vi "Spectrometer - Test activeX.vi"() -> ()   [LabVIEW 2014]
uses:
  NGSLabspec/NGSLabSpec.llb/MoveMotor Mode.ctl
  NGSLabspec/NGSLabSpec.llb/MoveMotor Motor Name.ctl
  NGSLabspec/NGSLabSpec.llb/GetMotorPosition Mode.ctl
  NGSLabspec/NGSLabSpec.llb/Acquire Mode.ctl
  NGSLabspec/NGSLabSpec.llb/GetValue Mode.ctl
  NGSLabspec/NGSLabSpec.llb/PutValue Name.ctl
  NGSLabspec/NGSLabSpec.llb/Template Mode.ctl
  NGSLabspec/NGSLabSpec.llb/Template Parameter.ctl
  NGSLabspec/NGSLabSpec.llb/GetMotorPosition Label Option.ctl
  NGSLabspec/NGSLabSpec.llb/Exec Command.ctl
panel:
  in  "stop":bool
  in  "OK Button":bool
  out "DataID":i32
  in  "Function":T1(tab)
  out "Array":i32[](array[numeric])
  in  "GetValue Mode":T2
  out "Value":variant
  in  "pValue":variant
  in  "Name":T3
  in  "Acquisition Mode":T4 items=["Spectrum", "Image", "Spectrum (Labspec Parameters)", "Spectral Image", "Get Detector Temperature", "Real Time Acquisition", "Set Photomultiplier Parameter", "Macro Spot", "Cancel Acquisition", "Set Detector"]
  in  "From (nm)":dbl=1.0
  in  "To (nm)":dbl=1.0
  in  "Integration Time (s)":dbl=1.0
  in  "Number of Accumulations":i32
  out "Acq":i32
  in  "Mode":T5 items=["Value"=0, "Step"=1, "Index"=2, "String"=3, "Calibrate"=4, "Origin"=5, "Stop"=6, "Value to Step"=7, "No Wait"=10, "No Message"=100]
  in  "Motor Name":T6=enum."Hole"
  in  "Position Value":dbl=1.0
  in  "Position Name":string
  out "MoveID":i32
  in  "Mode":T7 items=["Value", "Step", "Index", "Size", "Full Size"]
  in  "Motor Name":T6
  out "Position":string
  in  "Label Option":T8 items=[""=0, "Index to Value"=10, "Index to String"=20, "Full Index to Value"=30, "Full Index to String"=40]
  out "pValue Out":variant
  in  "Template Mode":T9
  in  "Template Parameter":T10
  in  "Template Name":string
  in  "Template Value":variant
  out "error out":errorcluster
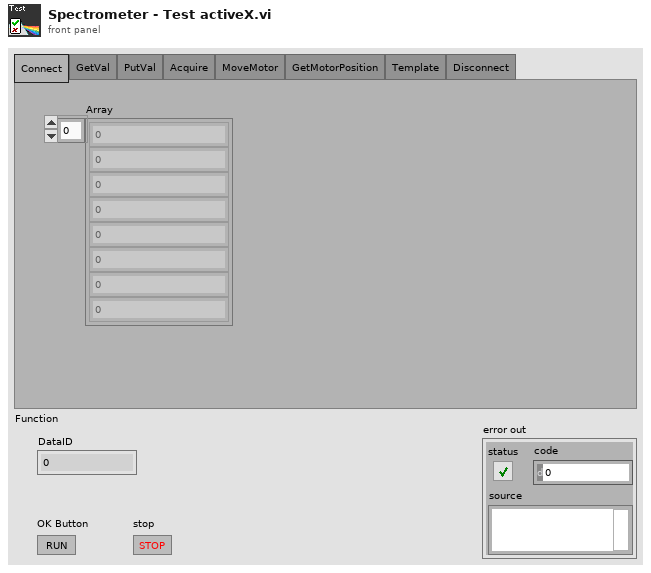
[diagram p1: front panel]
types:
  T1 = enum32{"Connect", "GetVal", "PutVal", "Acquire", "MoveMotor", "GetMotorPosition", "Template", "Disconnect"}
  T2 = typedef "GetValue Mode.ctl" = enum16{"XY Data", "Data", "MapPoint: Spectrum Index", "Axis Labels", "Axis Units", "Axis", "Axis Index", "Axis Size", "Axis Type", "Intensity", "Frequency", "X", "Y", "Z", "Time", "Double Cursor", "Pointer Limits", "Active Cursors", "Nearest Axis Index", "Acquisition Information", "Custom Information", "History Information", "Data Name", "Dispersion", "Dispersion Parameters", "Labspec Path", "User Level", "System Name", "Autofocus Diode", "Exposure Time", "Live Time", "Labspec Accumulation", "Alignment Diode"}
  T3 = typedef "PutValue Name.ctl" = enum16{"XY Data", "Data", "MapPoint:SpectrumIndex", "Axis Labels", "Axis Units", "Axis", "Axis Limits", "Frequency Unit", "Intensity Unit", "Cursor Type", "Pointer Limits", "Active Cursors", "Special Script Type", "CCD Shutter", "Laser", "SWIFT", "Labspec Exposure Time", "Labspec Accumulation", "Active Frame"}
  T4 = typedef "Acquire Mode.ctl" = u16
  T5 = typedef "MoveMotor Mode.ctl" = u16
  T6 = typedef "MoveMotor Motor Name.ctl" = enum16{"Spectro", "Premono", "Grating", "Slit", "Hole", "X", "Y", "XT", "YT", "XL", "YL", "Z", "Laser", "Filter", "Objective", "Detector", "Detector Temperature"}
  T7 = typedef "GetMotorPosition Mode.ctl" = u16
  T8 = typedef "GetMotorPosition Label Option.ctl" = u16
  T9 = typedef "Template Mode.ctl" = enum16{"Load", "Save", "Add To List", "Set Value", "Get Value", "Apply ", "Get Status", "Save Current Config", "Test", "Apply No Spectro"}
  T10 = typedef "Template Parameter.ctl" = enum16{"Laser", "Filter", "Accumulation", "Spike", "Auto Exposure", "Auto Focus", "Grating", "Raman Polarizer", "Laser Polarizer", "Central Position", "Position From", "Position To", "Exposition", "Hole", "Slit", "AutoExposure Min", "AutoExposure Max", "Extended Range", "Objective"}
  T11 = enum16{"Generic Data", "Spectrum", "Spectral Profile Image", "Map", "Video", "First Data", "Next Data"}
  T12 = typedef "Exec Command.ctl" = u16
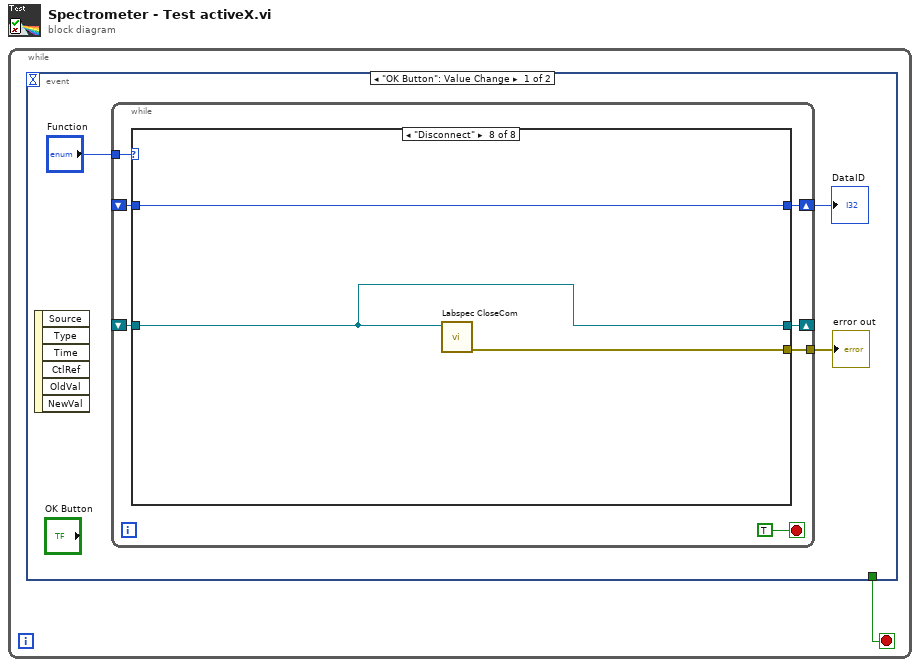
[diagram p0: block diagram]
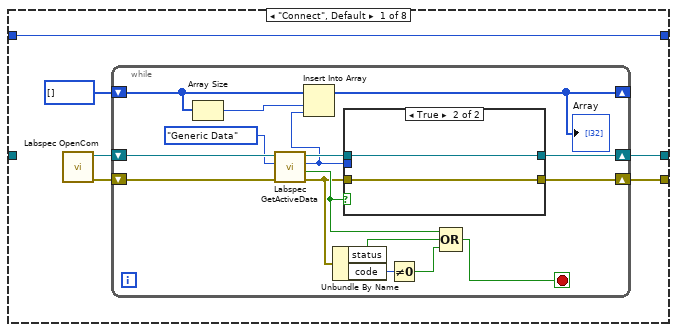
[diagram p2: hidden frame]
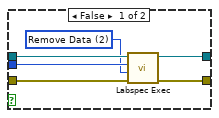
[diagram p3: hidden frame]
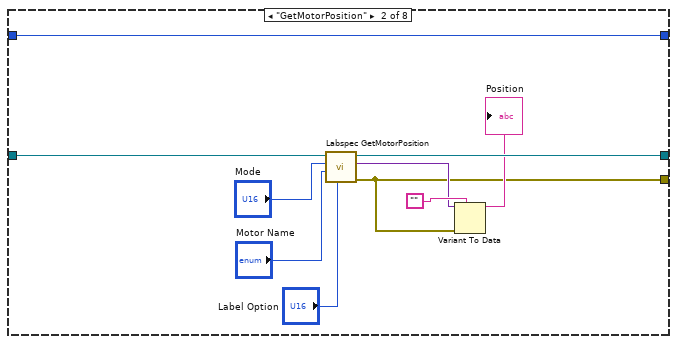
[diagram p4: hidden frame]
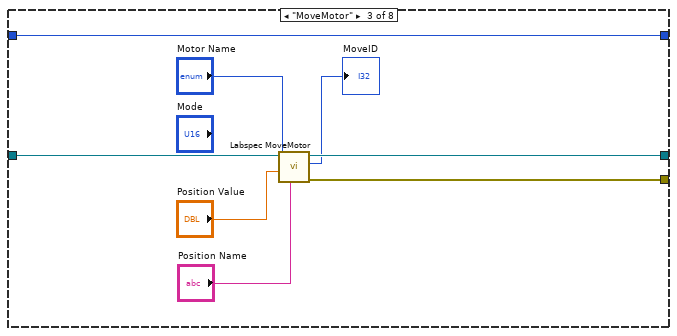
[diagram p5: hidden frame]
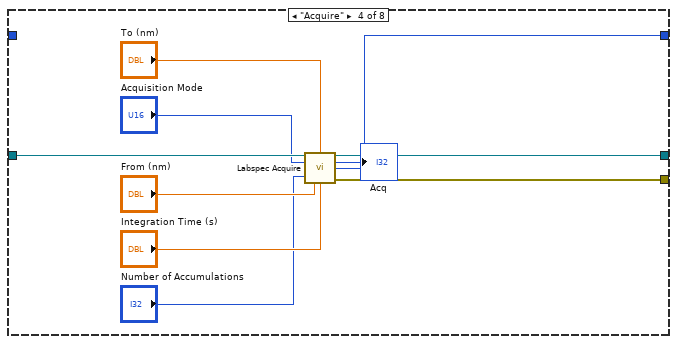
[diagram p6: hidden frame]
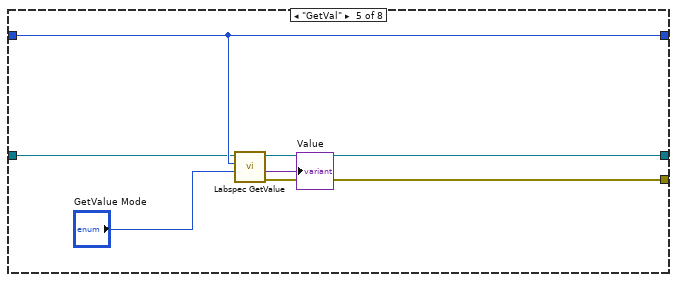
[diagram p7: hidden frame]
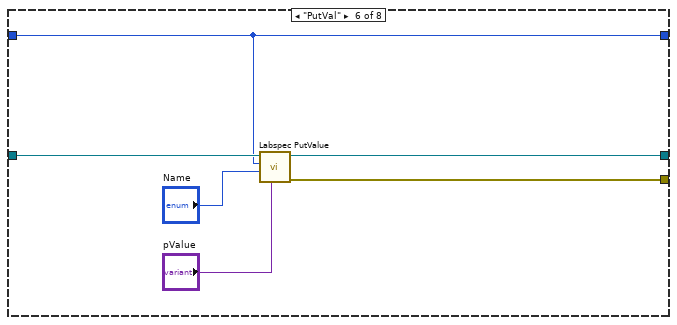
[diagram p8: hidden frame]
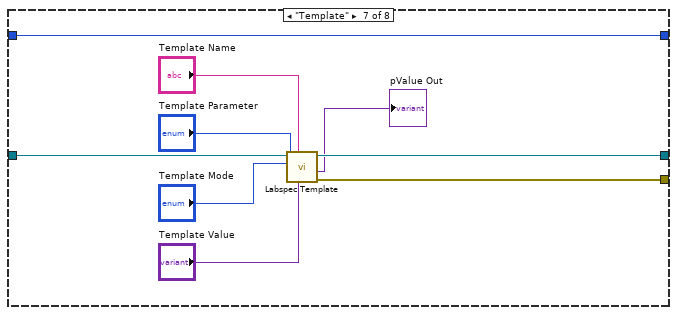
[diagram p9: hidden frame]
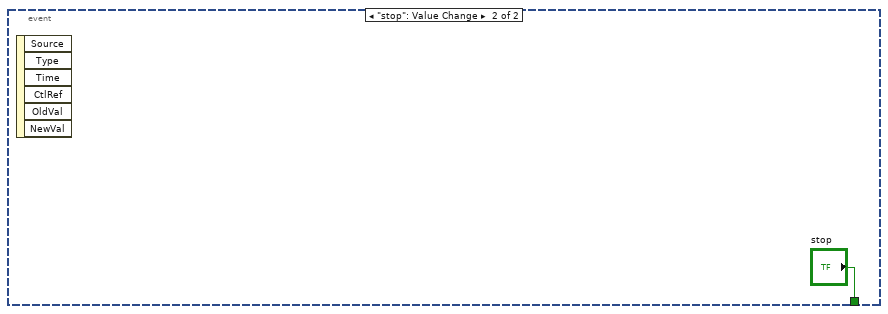
[diagram p10: hidden frame]
diagram:
  n1 = while {
    stop <- w1 stop-if-true
    n2 = event shown="[0] \"OK Button\": Value Change" {
      selector: _ -> [_ _]
      dyn-events: _ -> [_ _]
      timeout: _ -> [_ _]
      tunnel: [_ "stop"] -> w1
      event "OK Button": Value Change {
        n3 = event-data() -> ()  [unwired: 1 in, 6 out]
        n4 = while {
          shift-right: [w11] -> _
          shift-left: _ -> [w9]
          tunnel: [w10] -> w4
          tunnel: "Function" -> [w7]
          shift-right: [w6] -> w2
          shift-left: _ -> [w5]
          stop <- TRUE stop-if-true
          n5 = case shown="\"Disconnect\"" w7 {
            tunnel: [w14 w50 w58 w68 w71 w80 w87 w93] -> w11
            tunnel: [w13 w42 w57 w67 w74 w79 w89 w92] -> w10
            tunnel: w9 -> [_ w51 w59 w69 w72 w81 w88 w93]
            tunnel: [w17 w47 w52 w61 w75 w78 w90 w91] -> w6
            tunnel: w5 -> [w17 w47 w52 _ w75 w78 w90 w91]
            frame "Connect", Default {
              n6 = call "Labspec OpenCom.vi"() -> ("error out"=w15:errorcluster, "Automation Refnum"=w16:refnum<k7>)  [unwired: 1 in, 9 out]
              n7 = while {
                shift-right: [w30] -> w14
                shift-left: w16 -> [w32]
                shift-right: [w29] -> w13
                shift-left: w15 -> [w31]
                shift-right: [w18] -> _
                shift-left: i32[] [] -> [w20]
                stop <- w22 stop-if-true
                n8 = Array Size(array=w20) -> (size(s)=w19:i32)
                n9 = call "Labspec GetActiveData.vi"("error in"=w31, "Data Type"=T11."Generic Data", "Automation Refnum In"=w32) -> ("error out"=w26:errorcluster, "No Active Data?"=w27:bool, "Data ID"=w21:i32, "Automation Refnum Out"=w33:refnum<k7>)  [unwired: 5 in]
                n10 = Insert Into Array(array=w20, index=w19, new element=w21) -> (w18:i32[])
                "Array" <- w18
                n11 = Unbundle By Name(w26) -> ("status"=w25:bool, "code"=w24:i32)
                n12 = case shown="True" w27 {
                  tunnel: w33 -> [w39 w41]
                  tunnel: w26 -> [w38 w40]
                  tunnel: [w37 w41] -> w30
                  tunnel: [w36 w40] -> w29
                  tunnel: w21 -> [w35 _]
                  frame False {
                    w34 = T12 2 items=["Show data", "Hide data", "Remove Data", "Clone Data", "Show Style", "Show Mode", "Show Axis", "Hide all"] ("Command")
                    n13 = call "Labspec Exec.vi"("error in"=w38, "Command"=w34, "Data ID"=w35, "Automation Refnum In"=w39) -> ("error out"=w36:errorcluster, "Automation Refnum Out"=w37:refnum<k7>)  [unwired: 4 in, 2 out]
                  }
                  frame True {
                  }
                }
                n14 = Not Equal To 0?(x=w24) -> (x != 0?=w23:bool)
                n15 = Compound Arithmetic op=OR(w27, w25, w23) -> (w22:bool)
              }
            }
            frame "GetMotorPosition" {
              n16 = call "Labspec GetMotorPosition.vi"("Label Option"="Label Option", "Motor Name"="Motor Name", "Mode"="Mode", "Automation Refnum In"=w51) -> ("error out"=w42:errorcluster, "Position"=w44:variant, "Automation Refnum Out"=w50:refnum<k7>)  [unwired: 1 in, 4 out]
              n17 = Variant To Data(error in=w42, type="", Variant=w44) -> (data=→"Position":string)  [unwired: 1 out]
            }
            frame "MoveMotor" {
              n18 = call "Labspec MoveMotor.vi"("Position Name"="Position Name", "Position Value"="Position Value", "Motor Name"="Motor Name", "Automation Refnum In"=w59) -> ("error out"=w57:errorcluster, "MoveID"=→"MoveID":i32, "Automation Refnum Out"=w58:refnum<k7>)  [unwired: 5 in]
            }
            frame "Acquire" {
              n19 = call "Labspec Acquire.vi"("Automation Refnum In"=w69, "From (nm)"="From (nm)", "To (nm)"="To (nm)", "Mode"="Acquisition Mode", "Number of Accumulations"="Number of Accumulations", "Integration Time (s)"="Integration Time (s)") -> ("Automation Refnum Out"=w68:refnum<k7>, "Acq"=→"Acq":i32, "AcqID"=w61:i32, "error out"=w67:errorcluster)  [unwired: 6 in]
            }
            frame "GetVal" {
              n20 = call "Labspec GetValue.vi"("GetValue Mode"="GetValue Mode", "DataID"=w75, "Automation Refnum In"=w72) -> ("error out"=w74:errorcluster, "pValue"=→"Value":variant, "Automation Refnum Out"=w71:refnum<k7>)  [unwired: 2 in, 4 out]
            }
            frame "PutVal" {
              n21 = call "Labspec PutValue.vi"("pValue"="pValue", "Name"="Name", "DataID"=w78, "Automation Refnum In"=w81) -> ("error out"=w79:errorcluster, "Automation Refnum Out"=w80:refnum<k7>)  [unwired: 1 in, 5 out]
            }
            frame "Template" {
              n22 = call "Labspec Template.vi"("Value"="Template Value", "Template Name"="Template Name", "Parameter"="Template Parameter", "Mode"="Template Mode", "Automation Refnum In"=w88) -> ("error out"=w89:errorcluster, "pValue"=→"pValue Out":variant, "Automation Refnum Out"=w87:refnum<k7>)  [unwired: 4 in]
            }
            frame "Disconnect" {
              n23 = call "Labspec CloseCom.vi"("Automation Refnum In"=w93) -> ("error out"=w92:errorcluster)  [unwired: 1 in, 9 out]
            }
          }
        }
        "error out" <- w4
        "DataID" <- w2
      }
      event "stop": Value Change {
        n24 = event-data() -> ()  [unwired: 1 in, 6 out]
      }
    }
  }
